vi "ApplyVisOptions.vi"(7 "section (optional)":string="Logging and Visualization", 8 "error in (no error)":errorcluster, 11 "INIFilePath":path) -> (0 "error out":errorcluster, 2 "VisualizationProperties":T1={"PauseAtStartup"=TRUE, "LogData"=FALSE, "LaunchInSubPanel"=TRUE, "FPMonitor"=0, "FPWindowBounds"={"Left"=0, "Top"=0, "Right"=0, "Bottom"=0}, "MonitorBounds"={"Left"=0, "Top"=0, "Right"=0, "Bottom"=0}, "MeasIndices"=[]})   [LabVIEW 2018, in "Visualization.lvlib" / "VisualizeStatus.lvclass"]
uses:
  StatusAndLog/VisualizeStatus.lvclass
  VisualizationOptions.ctl
  <vilib>/Utility/miscctls.llb/LVRectTypeDef.ctl
  VisualizeBase.lvclass
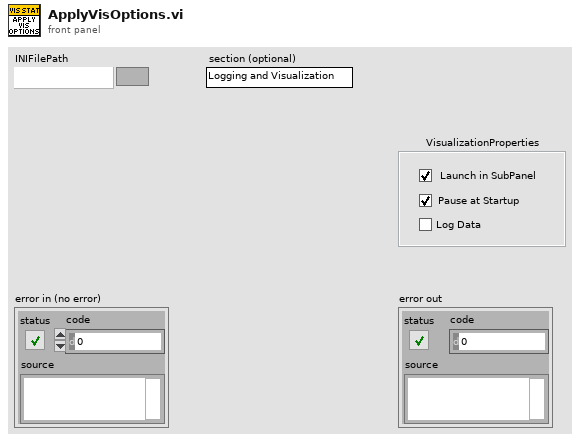
[diagram p1: front panel]
types:
  T1 = typedef "Visualization.lvlib/VisualizeBase.lvclass/VisualizationOptions.ctl" = cluster{"PauseAtStartup":bool, "LogData":bool, "LaunchInSubPanel":bool, "FPMonitor":u16, "FPWindowBounds":T2, "MonitorBounds":cluster{"Left":i16, "Top":i16, "Right":i16, "Bottom":i16}, "MeasIndices":i32[]}
  T2 = typedef "LVRectTypeDef.ctl" = cluster{"Left":i16, "Top":i16, "Right":i16, "Bottom":i16}
  T3 = cluster{"Left":i16, "Top":i16, "Right":i16, "Bottom":i16}
  T4 = typedef "LVAllMonitorsDisplayTypeDef.ctl" = cluster{"Bounds":cluster{"Left":i16, "Top":i16, "Right":i16, "Bottom":i16}, "Depth":i16}[]
  T5 = cluster{"Bounds":cluster{"Left":i16, "Top":i16, "Right":i16, "Bottom":i16}, "Depth":i16}
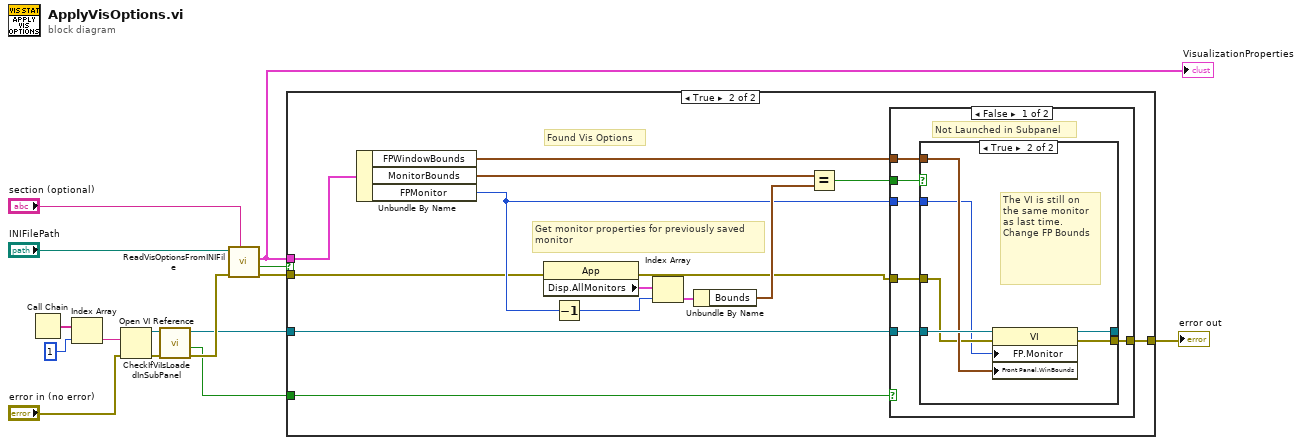
[diagram p0: block diagram]
diagram:
  n1 = Call Chain() -> (call chain=w5:string[])
  n2 = Index Array(array=w5, index=1) -> (element=w6:string)
  n3 = Open VI Reference(vi path=w6, error in (no error)="error in (no error)") -> (vi reference=w3:refnum<vi>, error out=w1:errorcluster)  [unwired: 4 in]
  n4 = call "CheckIfViIsLoadedInSubPanel.vi"("error in (no error)"=w1, "vi reference"=w3) -> ("error out"=w15:errorcluster, "In SubPanel?"=w8:bool, "VI reference out"=w9:refnum<vi>)  [unwired: 7 in]
  n5 = call "ReadVisOptionsFromINIFile.vi"("section (optional)"="section (optional)", "error in (no error)"=w15, "INI File Path"="INIFilePath") -> ("error out"=w12:errorcluster, "all found?"=w13:bool, "Visualization Properties"=w14:T1)  [unwired: 6 in]
  "VisualizationProperties" <- w14
  n6 = case shown="True" w13 {
    tunnel: w8 -> [_ w30]
    tunnel: w12 -> [w16 w17]
    tunnel: w14 -> [_ w29]
    tunnel: w9 -> [_ w28]
    tunnel: [w16 w27] -> w7
    frame False {
    }
    frame True {
      # "Get monitor properties for previously saved\nmonitor"
      # "Found Vis Options"
      n7 = Unbundle By Name(w29) -> ("FPWindowBounds"=w20:T2, "MonitorBounds"=w23:T3, "FPMonitor"=w18:u16)
      n8 = property class="App"(error in=w17) -> (error out=w19:errorcluster, "Disp.AllMonitors"=w26:T4)  [unwired: 1 in, 1 out]
      n9 = Decrement(x=w18) -> (x-1=w25:u16)
      n10 = Index Array(array=w26, index=w25) -> (element=w24:T5)
      n11 = Unbundle By Name(w24) -> ("Bounds"=w22:T3)
      n12 = Equal?(x=w23, y=w22) -> (x = y?=w21:bool)
      n13 = case shown="False" w30 {
        tunnel: w21 -> [w36 _]
        tunnel: w20 -> [w35 _]
        tunnel: w19 -> [w34 w45]
        tunnel: w28 -> [w33 _]
        tunnel: [w32 w45] -> w27
        tunnel: w18 -> [w31 _]
        frame False {
          # "Not Launched in Subpanel"
          n14 = case shown="True" w36 {
            tunnel: w33 -> [w38 w44]
            tunnel: w35 -> [_ w43]
            tunnel: w34 -> [w37 w42]
            tunnel: [w38 w41] -> _
            tunnel: [w37 w40] -> w32
            tunnel: w31 -> [_ w39]
            frame False {
            }
            frame True {
              # "The VI is still on the same monitor as last time. Change FP Bounds"
              n15 = property class="VI"(reference=w44, error in=w42, "FP.Monitor"=w39, "Front Panel.WinBounds"=w43) -> (reference out=w41:refnum<vi>, error out=w40:errorcluster)
            }
          }
        }
        frame True {
          # "Don't mess with FP Bounds if launched in sub panel"
        }
      }
    }
  }
  "error out" <- w7
